vi "SetDestinationFolder.vi"(8 "error in":errorcluster, 10 "DestinationFolder":path, 11 "Datawarehouse in":refnum<class "Datawarehouse.lvclass">) -> (0 "error out":errorcluster, 3 "Datawarehouse out":refnum<class "Datawarehouse.lvclass">)   [LabVIEW 2021, in "ProligentXMLGenerator.lvlib" / "Datawarehouse.lvclass"]
doc: "Absolute destination folder path."
uses:
  Datawarehouse.lvclass
  Datawarehouse.lvclass/Datawarehouse.ctl
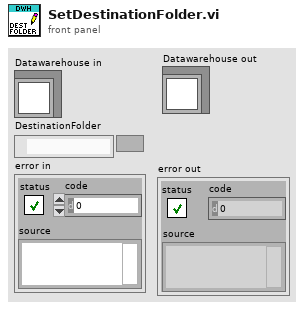
[diagram p1: front panel]
types:
  T1 = typedef "ProligentXMLGenerator.lvlib/Datawarehouse.lvclass/Data.ctl" = cluster{"DestinationFolder":path, "BaseFileName":string, "Document":refnum<k20>, "Defects":refnum<class "Defect.lvclass">[], "TopProcessRuns":refnum<class "ProcessRun.lvclass">[], "ProductUnits":refnum<class "ProductUnit.lvclass">[], "GenerationTime":refnum<class "DateTime.lvclass">, "DataSourceFingerprint":refnum<class "NonEmptyString_448.lvclass">, "IntegrationMetaData":refnum<class "NonEmptyString_2000.lvclass">, "TimeZoneInfoId":string}
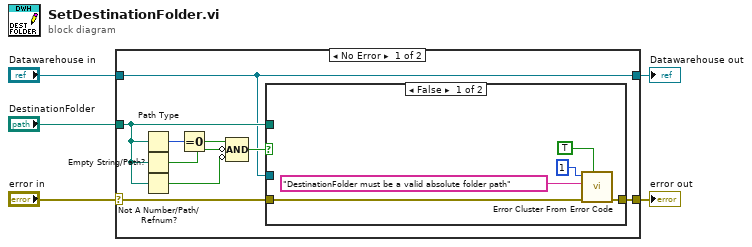
[diagram p0: block diagram]
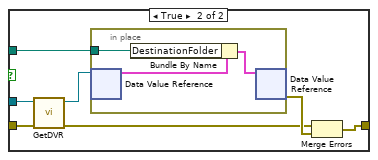
[diagram p2: hidden frame]
diagram:
  n1 = case shown="No Error" "error in" {
    selector: "error in" -> [w14 w30]
    tunnel: "Datawarehouse in" -> [w7 w31]
    tunnel: [w13 w30] -> w3
    tunnel: "DestinationFolder" -> [w9 _]
    tunnel: [w7 w31] -> w1
    frame No Error {
      n2 = Path Type(1:w9) -> (0:w12:i16)
      n3 = Empty String/Path?(string/path=w9) -> (empty?=w11:bool)
      n4 = Not A Number/Path/Refnum?(number/path/refnum=w9) -> (NaN/Path/Refnum?=w6:bool)
      n5 = Equal To 0?(x=w12) -> (x = 0?=w10:bool)
      n6 = Compound Arithmetic op=AND(w10, invert w11, invert w6) -> (w8:bool)
      n7 = case shown="False" w8 {
        tunnel: w14 -> [w15 w26]
        tunnel: w7 -> [_ w25]
        tunnel: [w18 w24] -> w13
        tunnel: w9 -> [_ w20]
        frame False {
          n8 = call <vilib>:"Error Cluster From Error Code.vi"("show call chain? (False)"=TRUE, "error in (no error)"=w15, "error message (\"\")"="DestinationFolder must be a valid absolute folder path", "error code (0)"=1) -> ("error out"=w18:errorcluster)  [unwired: 5 in]
        }
        frame True {
          n9 = call "GetDVR.vi"("error in"=w26, "Datawarehouse"=w25) -> ("error out"=w21:errorcluster, "DVRReference"=w22:refnum<data-value>)  [unwired: 8 in]
          n10 = in-place "In Place Element Structure" {
            in-place-border: w20 -> [w28]
            n11 = in-place-dvr #1(w22) -> (w27:T1)  [unwired: 1 out]
            n12 = Bundle By Name(cluster=w27, "DestinationFolder"=w28) -> (w29:T1)
            n13 = in-place-dvr #1(w29) -> (w23:errorcluster)  [unwired: 1 out]
          }
          n14 = Merge Errors(w21, w23) -> (w24:errorcluster)
        }
      }
    }
    frame Error {
    }
  }
  "error out" <- w3
  "Datawarehouse out" <- w1
